vi "NextGoal.vi"(10 "Goal list":cluster{"X":sgl, "Y":sgl, "theta":dbl}[](array[cluster]), 11 "Current Index":i32) -> (1 "Finish track?":bool, 2 "Next Goal":cluster{"X":sgl, "Y":sgl, "theta":dbl}, 3 "Goal Index":i32)   [LabVIEW 2016]
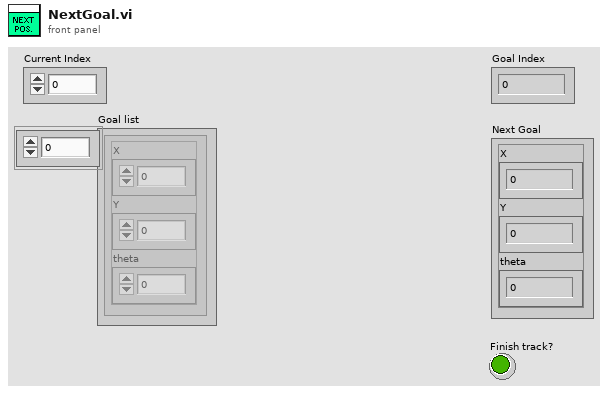
[diagram p1: front panel]
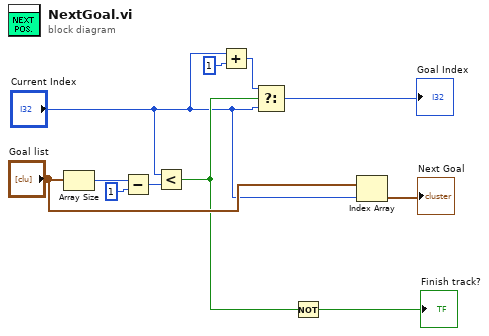
[diagram p0: block diagram]
diagram:
  n1 = Array Size(array="Goal list") -> (size(s)=w7:i32)
  n2 = Subtract(x=w7, y=1) -> (x-y=w8:i32)
  n3 = Less?(x="Current Index", y=w8) -> (x < y?=w3:bool)
  n4 = Add(x="Current Index", y=1) -> (x+y=w10:i32)
  n5 = Select(t=w10, s=w3, f="Current Index") -> (s? t:f=→"Goal Index":i32)
  n6 = Not(x=w3) -> (.not. x?=→"Finish track?":bool)
  n7 = Index Array(array="Goal list", index="Current Index") -> (element=→"Next Goal":cluster{"X":sgl, "Y":sgl, "theta":dbl})
